vi "Edit Connector Pane for wrapper.vi"(0 "vi reference":refnum<vi>, 11 "error in (no error)":errorcluster) -> (4 "vi reference out":refnum<vi>, 15 "error out":errorcluster)   [LabVIEW 2021, in "Migrator.lvlib"]
uses:
  Migrator.lvlib
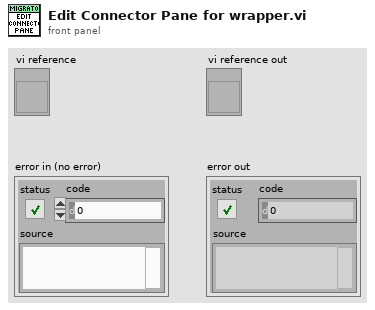
[diagram p1: front panel]
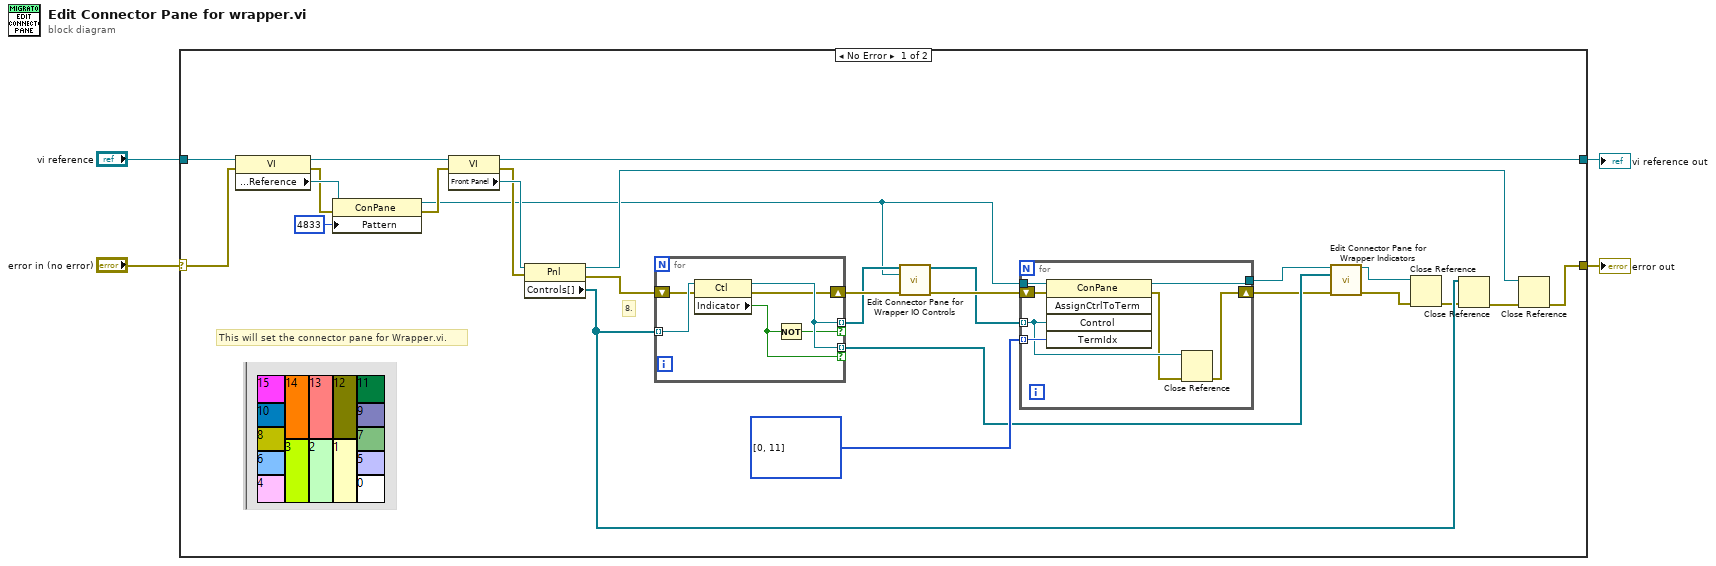
[diagram p0: block diagram]
diagram:
  n1 = case shown="No Error" "error in (no error)" {
    selector: "error in (no error)" -> [w19 w46]
    tunnel: [w14 w46] -> w4
    tunnel: "vi reference" -> [w12 w45]
    tunnel: [w11 w45] -> w1
    frame No Error {
      # "8."
      # "This will set the connector pane for Wrapper.vi."
      n2 = property class="VI"(reference=w12, error in=w19) -> (reference out=w31:refnum<vi>, error out=w26:errorcluster, "Connector Pane:Reference"=w28:refnum<vi>)
      n3 = property class="ConPane"(reference=w28, error in=w26, "Pattern"=u32 4833) -> (reference out=w6:refnum<vi>, error out=w27:errorcluster)
      n4 = property class="VI"(reference=w31, error in=w27) -> (reference out=w11:refnum<vi>, error out=w29:errorcluster, "Front Panel"=w30:refnum<vi>)
      n5 = property class="Pnl"(reference=w30, error in=w29) -> (reference out=w18:refnum<vi>, error out=w10:errorcluster, "Controls[]"=w17:refnum<vi>[])
      n6 = for {
        tunnel: w17 -> [w37] mode=indexing
        shift-right: [w32] -> w9
        shift-left: w10 -> [w36]
        tunnel: [w35] -> w22 mode=indexing if=w34
        tunnel: [w35] -> w7 mode=indexing if=w33
        n7 = property class="Ctl"(reference=w37, error in=w36) -> (reference out=w35:refnum<vi>, error out=w32:errorcluster, "Indicator"=w34:bool)
        n8 = Not(x=w34) -> (.not. x?=w33:bool)
      }
      n9 = call "Edit Connector Pane for Wrapper IO Controls.vi"("ControlsIn[]"=w7, "ConPaneIn"=w6, "error in"=w9) -> ("OtherControls[]"=w5:refnum<vi>[], "error out"=w8:errorcluster)  [unwired: 11 in]
      n10 = for {
        tunnel: w5 -> [w40] mode=indexing
        tunnel: u32[] [0, 11] ("Terminal Index") -> [w44] mode=indexing
        tunnel: w6 -> [w43]
        shift-right: [w38] -> w21
        shift-left: w8 -> [w42]
        tunnel: [w41] -> w24
        n11 = invoke class="ConPane" method="AssignCtrlToTerm"(reference=w43, error in=w42, "Control"=w40, "TermIdx"=w44) -> (reference out=w41:refnum<vi>, error out=w39:errorcluster)  [unwired: 1 in, 3 out]
        n12 = Close Reference(reference=w40, error in (no error)=w39) -> (error out=w38:errorcluster)
      }
      n13 = call "Edit Connector Pane for Wrapper Indicators.vi"("ConPaneIn"=w24, "IndicatorsIn[]"=w22, "error in"=w21) -> ("ConPaneOut"=w23:refnum<vi>, "error out"=w20:errorcluster)  [unwired: 11 in]
      n14 = Close Reference(reference=w23, error in (no error)=w20) -> (error out=w16:errorcluster)
      n15 = Close Reference(reference=w17, error in (no error)=w16) -> (error out=w15:errorcluster)
      n16 = Close Reference(reference=w18, error in (no error)=w15) -> (error out=w14:errorcluster)
    }
    frame Error {
    }
  }
  "error out" <- w4
  "vi reference out" <- w1
